vi "Set Power.vi"(7 "Correlation ID":u32, 8 "error in (no error)":errorcluster, 9 "Power":dbl, 11 "Laser Quantum in":refnum<class "Laser.lvclass">) -> (0 "error out":errorcluster, 3 "Laser Quantum out":refnum<class "Laser.lvclass">)   [LabVIEW 2023, in "Laser.lvlib" / "Laser.lvclass"]
uses:
  Laser.lvclass
  C:/Program Files/National Instruments/LabVIEW 2023/vi.lib/ActorFramework/Actor/Actor.lvclass
  <vilib>/ActorFramework/Actor/Actor.lvclass/Actor.ctl
  Application Messages/Set Laser Power Reply Msg/Set Laser Power Reply Msg.lvclass/Set Laser Power Reply Msg.ctl
  <vilib>/ActorFramework/Message Enqueuer/Message Enqueuer.lvclass/Message Enqueuer.ctl
  <vilib>/ActorFramework/Message Enqueuer/Enqueue.vi
  Application Messages/Set Laser Power Reply Msg/Set Laser Power Reply Msg.lvclass
  C:/Program Files/National Instruments/LabVIEW 2023/vi.lib/ActorFramework/Message/Message.lvclass
  <vilib>/ActorFramework/Message Priority Queue/Priority Enqueue.vi
  Laser.lvclass/Laser.ctl
  Application Messages/Automation_TaskCompleted Msg/Automation_TaskCompleted Msg.lvclass
  <vilib>/ActorFramework/Actor/Actor.lvclass
  C:/FlashGordon/Development/Hardware/Device/Device.lvclass
  C:/FlashGordon/Development/Hardware/Laser/Laser.lvclass
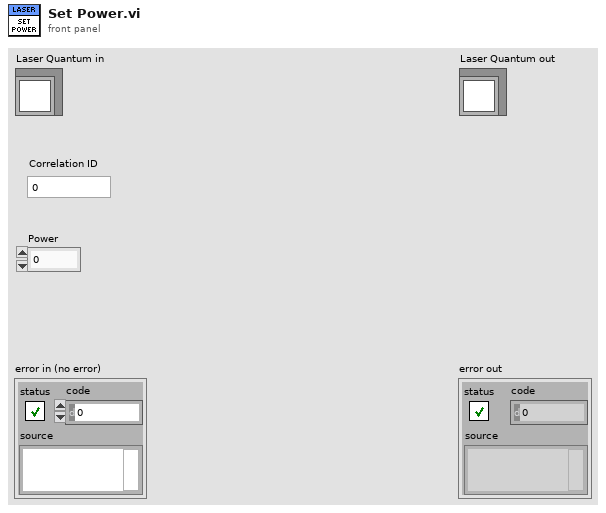
[diagram p1: front panel]
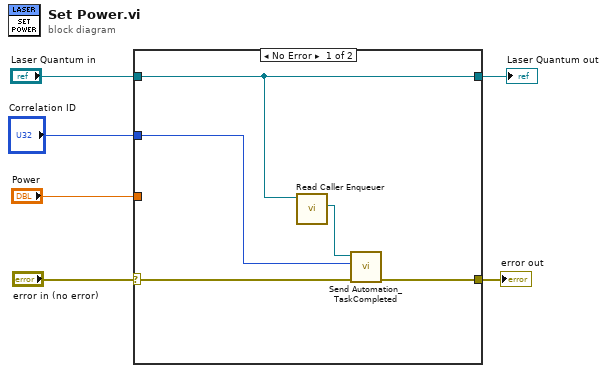
[diagram p0: block diagram]
diagram:
  n1 = case shown="No Error" "error in (no error)" {
    selector: "error in (no error)" -> [w11 w13]
    tunnel: [w10 w13] -> w5
    tunnel: [w9 w12] -> w3
    tunnel: "Laser Quantum in" -> [w9 w12]
    tunnel: "Power" -> [_ _]
    tunnel: "Correlation ID" -> [w7 _]
    frame No Error {
      n2 = call <vilib>:"Read Caller Enqueuer.vi"("Actor"=w9) -> ("Caller Enqueuer"=w8:refnum<class "Message Enqueuer.lvclass">)  [unwired: 10 in]
      n3 = call "Send Automation_TaskCompleted.vi"("error in (no error)"=w11, "Correlation ID"=w7, "Message Enqueuer"=w8) -> ("error out"=w10:errorcluster)  [unwired: 7 in, 1 out]
    }
    frame Error {
    }
  }
  "error out" <- w5
  "Laser Quantum out" <- w3
